vi "Module Loop.vi"(8 "error in (no error)":errorcluster, 11 "System Config Server in":refnum<class "System Config Module.lvclass">) -> (0 "error out":errorcluster, 3 "System Config Server out":refnum<class "System Config Module.lvclass">)   [LabVIEW 2020, in "Volatus.lvlib" / "System Config Module.lvclass"]
uses:
  System Config Module.lvclass
  C:/dev/lv20CE/relink/lv-volatus/Volatus/Module/Module.lvclass
  Module/Module.lvclass/Module.ctl
  MessageQ/MessageQ.lvclass/MessageQ.ctl
  Module/Module.lvclass
  New Config.ctl
  System Config Module.lvclass/System Config Module.ctl
  lv-cdm/CDM-Config/ISO8601 Config.ctl
  lv-cdm/CDM-Config/Format.ctl
  lv-cdm/CDM-Config/Precision.ctl
  lv-cdm/CDM-Config/Timezone.ctl
  VolatusConfig/Config Format.ctl
  Config Info.ctl
  ConfigInfoValue/ConfigInfoValue.lvclass/ConfigInfoValue.ctl
  Module/Self Q.vi
  MessageQ/Send.vi
  Module/Parent Q.vi
  <vilib>/AdvancedString/Delimited String to 1D String Array.vi
  <vilib>/dlg_ctls.llb/Space Constant.vi
  VolatusAPI/Build Node URL.vi
  <vilib>/httpClient/POSTMultipart.vi
  lv-cdm/CDM-Config/ISO-8601 Format Strings.vi
  <vilib>/Utility/error.llb/Error Cluster From Error Code.vi
  lv-promises/Promises/Promise/Promise.lvclass
  ConfigInfoValue/ConfigInfoValue.lvclass
  MessageQ/MessageQ.lvclass
  lv-builder/Builder Core/Builder Core.lvlib
  Volatus.lvlib
  VolatusAPI/VolatusAPI.lvclass
  lv-cdm/CDM-Config/CDM-Config.lvlib
  VolatusConfig/VolatusConfig.lvlib
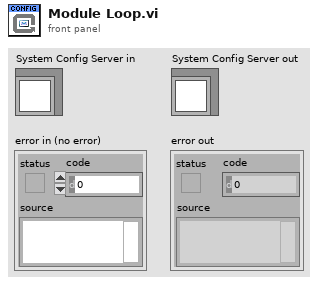
[diagram p1: front panel]
types:
  T1 = enum32{"Invalid", "Standard", "Closed", "Hidden", "Minimized", "Maximized"}
  T2 = typedef "Volatus.lvlib/New Config.ctl" = cluster{"System":string, "Cluster":string, "Node":string, "Config":string}
  T3 = enum16{"open", "replace", "create", "open or create", "replace or create", "replace or create with confirmation"}
  T4 = typedef "VolatusConfig.lvlib/Config Format.ctl" = enum16{"JSON", "INI", "SQLite"}
  T5 = typedef "CDM-Config.lvlib/ISO8601 Config.ctl" = cluster{"Format":T6, "Precision":T7, "Timezone":T8}
  T6 = typedef "CDM-Config.lvlib/Format.ctl" = enum16{"Extended", "Basic"}
  T7 = typedef "CDM-Config.lvlib/Precision.ctl" = enum16{"Millisecond", "Second", "Minute", "Hour", "Day"}
  T8 = typedef "CDM-Config.lvlib/Timezone.ctl" = enum16{"UTC", "Local"}
  T9 = typedef "Volatus.lvlib/Config Info.ctl" = cluster{"System":string, "Cluster":string, "Node":string, "Path":path, "Version":string, "Hash":string}
  T10 = typedef "Builder Core.lvlib/Version.ctl" = cluster{"Major":u16, "Minor":u16, "Fix":u16, "Build":u16}
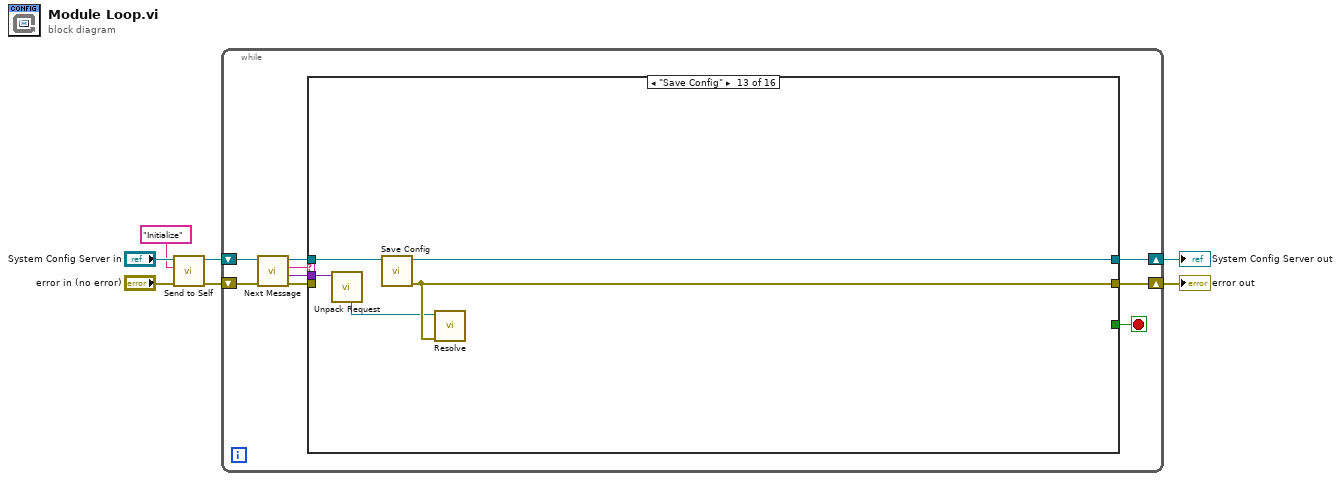
[diagram p0: block diagram]
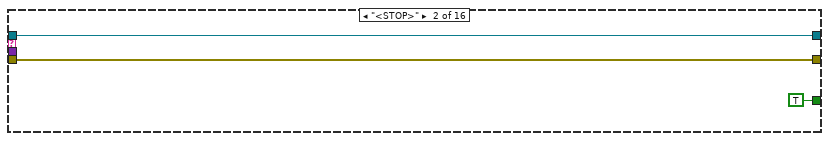
[diagram p3: hidden frame]
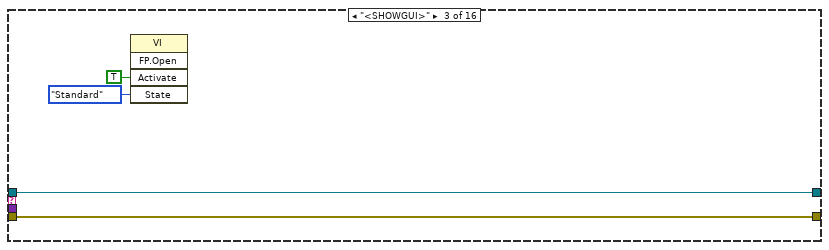
[diagram p4: hidden frame]
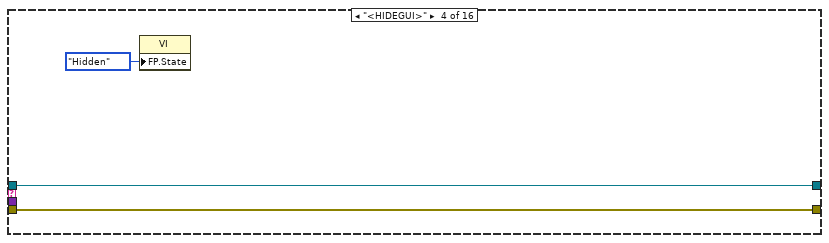
[diagram p5: hidden frame]
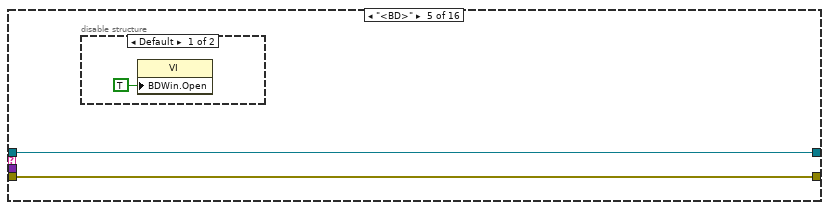
[diagram p6: hidden frame]
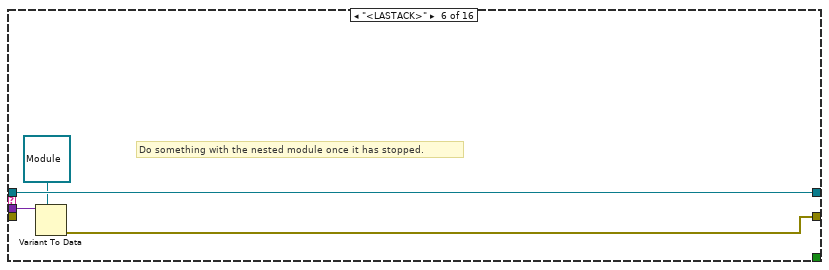
[diagram p8: hidden frame]
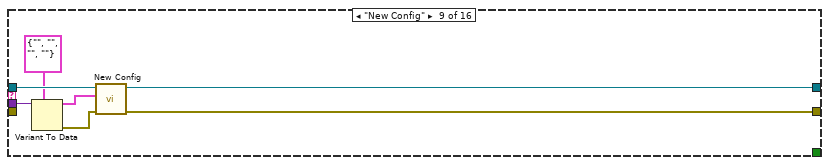
[diagram p11: hidden frame]
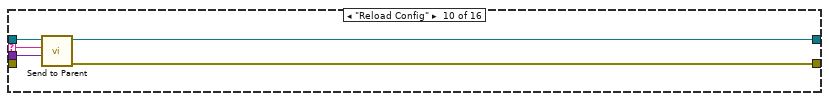
[diagram p12: hidden frame]
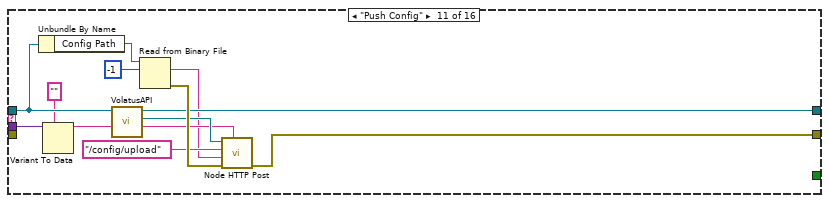
[diagram p13: hidden frame]
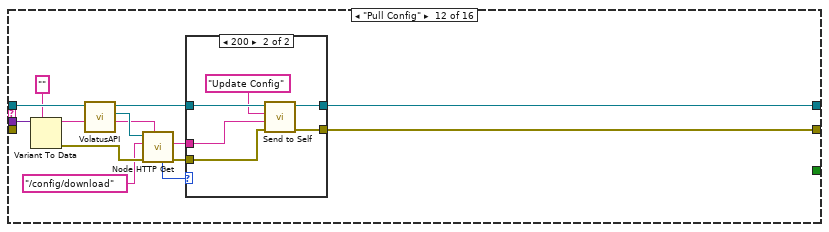
[diagram p14: hidden frame]
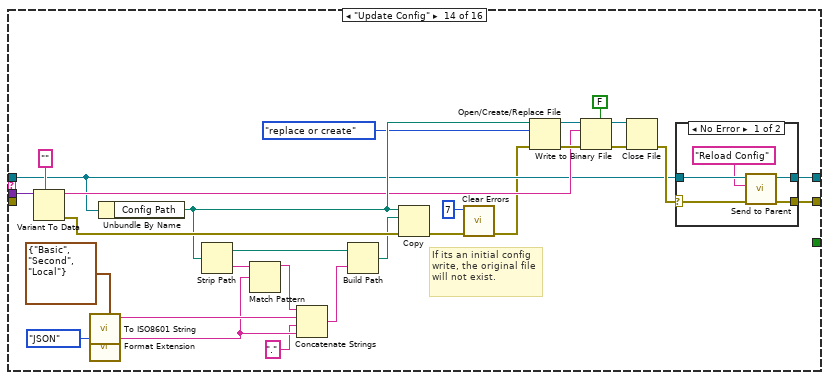
[diagram p16: hidden frame]
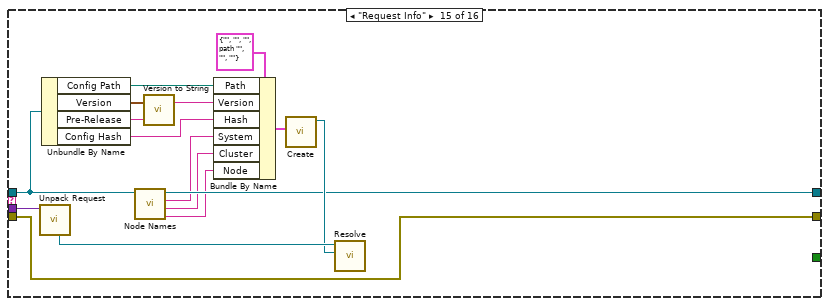
[diagram p18: hidden frame]
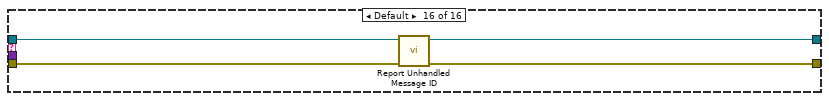
[diagram p19: hidden frame]
diagram:
  n1 = call "Send to Self.vi"("error in (no error)"="error in (no error)", "Message ID"="Initialize", "Module in"="System Config Server in") -> ("error out"=w4:errorcluster, "Module out"=w2:refnum<class "System Config Module.lvclass">)  [unwired: 7 in]
  n2 = while {
    shift-right: [w11] -> w6
    shift-left: w2 -> [w16]
    shift-right: [w8] -> w5
    shift-left: w4 -> [w15]
    stop <- w10 stop-if-true
    n3 = call "Next Message.vi"("error in (no error)"=w15, "Module in"=w16) -> ("error out"=w14:errorcluster, "Data"=w9:variant, "ID"=w13:string, "Module out"=w12:refnum<class "System Config Module.lvclass">)  [unwired: 6 in]
    n4 = case shown="\"Save Config\"" w13 {
      selector: w13 -> [_ _ _ _ _ _ _ _ _ w49 _ _ _ _ _ _]
      tunnel: w14 -> [w17 w19 w24 w27 w29 _ w36 w38 _ _ _ _ _ _ w125 w144]
      tunnel: w12 -> [w18 w21 w25 w28 w30 w35 w37 w39 w46 w51 w62 w75 w88 w92 w130 w142]
      tunnel: [w18 w21 w25 w28 w30 w35 w37 w39 w43 w50 w59 w68 w86 w94 w129 w141] -> w11
      tunnel: [_ TRUE _ _ _ _ _ _ _ _ _ _ _ _ _ _] -> w10
      tunnel: w9 -> [_ _ _ _ _ w34 _ _ w45 w48 w57 w74 w87 w115 w140 _]
      tunnel: [w17 w19 w24 w27 w29 w32 w36 w38 w40 w47 w52 w64 w89 w93 w125 w143] -> w8
      frame "<CLOSE>" {
      }
      frame "<STOP>" {
      }
      frame "<SHOWGUI>" {
        n5 = invoke class="VI" method="FP.Open"("Activate"=TRUE ("Activate?"), "State"=T1."Standard") -> ()  [unwired: 3 in, 5 out]
      }
      frame "<HIDEGUI>" {
        n6 = property class="VI"("FP.State"=T1."Hidden" ("Front Panel Window:State")) -> ()  [unwired: 2 in, 2 out]
      }
      frame "<BD>" {
        n7 = disable-structure shown="Default" {
          frame condition #0 (active) {
            n8 = property class="VI"("BDWin.Open"=TRUE ("Block Diagram Window:Open")) -> ()  [unwired: 2 in, 2 out]
          }
          frame condition #1 {
          }
        }
      }
      frame "<LASTACK>" {
        # "Do something with the nested module once it has stopped."
        n9 = Variant To Data(type=refnum<class "Module.lvclass"> refnum ("Volatus:Module"), Variant=w34) -> (error out=w32:errorcluster)  [unwired: 1 in, 1 out]
      }
      frame "<TIMEOUT>" {
        # "No message for this module was received in time"
      }
      frame "Initialize" {
      }
      frame "New Config" {
        n10 = Variant To Data(type=T2 {"System"="", "Cluster"="", "Node"="", "Config"=""} ("New Config"), Variant=w45) -> (data=w42:T2, error out=w41:errorcluster)  [unwired: 1 in]
        n11 = call "New Config.vi"("error in (no error)"=w41, "New Config"=w42, "System Config Module in"=w46) -> ("error out"=w40:errorcluster, "System Config Module out"=w43:refnum<class "System Config Module.lvclass">)  [unwired: 7 in]
      }
      frame "Reload Config" {
        n12 = call "Send to Parent.vi"("Data"=w48, "Message ID"=w49, "Module in"=w51) -> ("error out"=w47:errorcluster, "Module out"=w50:refnum<class "System Config Module.lvclass">)  [unwired: 7 in]
      }
      frame "Push Config" {
        n13 = Unbundle By Name(w62) -> ("Config Path"=w61:path)
        n14 = Variant To Data(type="", Variant=w57) -> (data=w55:string)  [unwired: 1 in, 1 out]
        n15 = call "VolatusAPI.vi"("Module in"=w62) -> ("VolatusAPI"=w58:refnum<class "VolatusAPI.lvclass">, "Module out"=w59:refnum<class "System Config Module.lvclass">)  [unwired: 9 in]
        n16 = Read from Binary File(10:-1 ("count (1)"), 11:w61) -> (0:w63:errorcluster, 2:w53:string)  [unwired: 4 in, 2 out]
        n17 = call "Node HTTP Post.vi"("Node Name"=w55, "error in (no error)"=w63, "Payload"=w53, "Path"="/config/upload", "VolatusAPI in"=w58) -> ("error out"=w52:errorcluster)  [unwired: 2 in, 4 out]
      }
      frame "Pull Config" {
        n18 = Variant To Data(type="", Variant=w74) -> (data=w70:string, error out=w76:errorcluster)  [unwired: 1 in]
        n19 = call "VolatusAPI.vi"("Module in"=w75) -> ("VolatusAPI"=w71:refnum<class "VolatusAPI.lvclass">, "Module out"=w72:refnum<class "System Config Module.lvclass">)  [unwired: 9 in]
        n20 = call "Node HTTP Get.vi"("Node Name"=w70, "error in (no error)"=w76, "Path"="/config/download", "VolatusAPI in"=w71) -> ("error out"=w65:errorcluster, "Response"=w67:string, "Status Code"=w66:u32)  [unwired: 3 in, 2 out]
        n21 = case shown="200" w66 {
          tunnel: w72 -> [w78 w84]
          tunnel: [w78 w83] -> w68
          tunnel: w67 -> [_ w81]
          tunnel: w65 -> [w77 w80]
          tunnel: [w77 w79] -> w64
          frame Default {
          }
          frame 200 {
            n22 = call "Send to Self.vi"("error in (no error)"=w80, "Data"=w81, "Message ID"="Update Config", "Module in"=w84) -> ("error out"=w79:errorcluster, "Module out"=w83:refnum<class "System Config Module.lvclass">)  [unwired: 6 in]
          }
        }
      }
      frame "Save Config" {
        n23 = call "Unpack Request.vi"("Request Data"=w87) -> ("Promise"=w85:refnum<class "Promise.lvclass">)  [unwired: 8 in, 2 out]
        n24 = call "Save Config.vi"("System Config Module in"=w88) -> ("error out"=w89:errorcluster, "System Config Module out"=w86:refnum<class "System Config Module.lvclass">)  [unwired: 9 in]
        n25 = call "Resolve.vi"("error in (no error)"=w89, "Promise in"=w85) -> ()  [unwired: 8 in, 2 out]
      }
      frame "Update Config" {
        # "If its an initial config write, the original file will not exist."
        n26 = Variant To Data(type="", Variant=w115) -> (data=w97:string, error out=w116:errorcluster)  [unwired: 1 in]
        n27 = call "To ISO8601 String.vi"("Format Config"=T5 {"Format"=enum."Basic", "Precision"=enum."Second", "Timezone"=enum."Local"}) -> ("ISO 8601"=w109:string)  [unwired: 10 in]
        n28 = call "Format Extension.vi"("Format"=Config_Format."JSON") -> ("Extension"=w108:string)  [unwired: 2 in]
        n29 = Unbundle By Name(w92) -> ("Config Path"=w103:path)
        n30 = Strip Path(path=w103) -> (stripped path=w106:path, name=w111:string)
        n31 = Match Pattern(string=w111, regular expression=w108) -> (before substring=w110:string)  [unwired: 1 in, 3 out]
        n32 = Concatenate Strings(w110, w109, ".", w108) -> (w105:string)
        n33 = Build Path(base path=w106, name or relative path=w105) -> (appended path=w104:path)
        n34 = Copy(8:w116, 10:w104, 11:w103) -> (0:w100:errorcluster)  [unwired: 2 in, 2 out]
        n35 = call <vilib>:"Clear Errors.vi"("error in (no error)"=w100, "specific error code to clear (0: all)"=7) -> ("error out"=w91:errorcluster)  [unwired: 4 in, 1 out]
        n36 = Open/Create/Replace File(file path (use dialog)=w103, error in=w91, operation (0:open)=T3."replace or create") -> (refnum out=w101:refnum<file>, error out=w99:errorcluster)  [unwired: 3 in, 1 out]
        n37 = Write to Binary File(file (use dialog)=w101, data=w97, error in=w99, 5:FALSE ("prepend array or string size? (T)")) -> (refnum out=w95:refnum<file>, error out=w96:errorcluster)  [unwired: 2 in, 1 out]
        n38 = Close File(refnum=w95, error in=w96) -> (error out=w117:errorcluster)  [unwired: 1 out]
        n39 = case shown="No Error" w117 {
          selector: w117 -> [w120 w124]
          tunnel: w92 -> [w122 w123]
          tunnel: [w121 w123] -> w94
          tunnel: [w119 w124] -> w93
          frame No Error {
            n40 = call "Send to Parent.vi"("error in (no error)"=w120, "Message ID"="Reload Config", "Module in"=w122) -> ("error out"=w119:errorcluster, "Module out"=w121:refnum<class "System Config Module.lvclass">)  [unwired: 7 in]
          }
          frame Error {
          }
        }
      }
      frame "Request Info" {
        n41 = call "Unpack Request.vi"("Request Data"=w140) -> ("Promise"=w132:refnum<class "Promise.lvclass">)  [unwired: 8 in, 2 out]
        n42 = Unbundle By Name(w130) -> ("Config Path"=w136:path, "Version"=w139:T10, "Pre-Release"=w138:string, "Config Hash"=w134:string)
        n43 = call "Node Names.vi"("Module in"=w130) -> ("Node"=w126:string, "Cluster"=w127:string, "System"=w128:string, "Module out"=w129:refnum<class "System Config Module.lvclass">)  [unwired: 6 in, 1 out]
        n44 = call "Version to String.vi"("Version"=w139, "Pre-Release (None)"=w138) -> ("Version String"=w135:string)  [unwired: 5 in]
        n45 = Bundle By Name(cluster=T9 {"System"="", "Cluster"="", "Node"="", "Path"=path "", "Version"="", "Hash"=""} ("Config Info"), "Path"=w136, "Version"=w135, "Hash"=w134, "System"=w128, "Cluster"=w127, "Node"=w126) -> (w133:T9)
        n46 = call "Create.vi"("Config Info"=w133) -> ("ConfigInfoValue out"=w131:refnum<class "ConfigInfoValue.lvclass">)  [unwired: 10 in]
        n47 = call "Resolve.vi"("Result (None)"=w131, "Promise in"=w132) -> ()  [unwired: 8 in, 2 out]
      }
      frame Default {
        n48 = call "Report Unhandled Message ID.vi"("error in (no error)"=w144, "Module in"=w142) -> ("error out"=w143:errorcluster, "Module out"=w141:refnum<class "System Config Module.lvclass">)  [unwired: 8 in]
      }
    }
  }
  "error out" <- w5
  "System Config Server out" <- w6
